vi "MCS.vi"(1 "MCS input":T1(array[cluster]) {"binning (s)" format="%.2f"; "binning (s)" format="%.2f"}, 2 "set":bool) -> (0 "MCS output":T1(array[cluster]) {"binning (s)" format="%.2f"; "binning (s)" format="%.2f"})   [LabVIEW 2009]
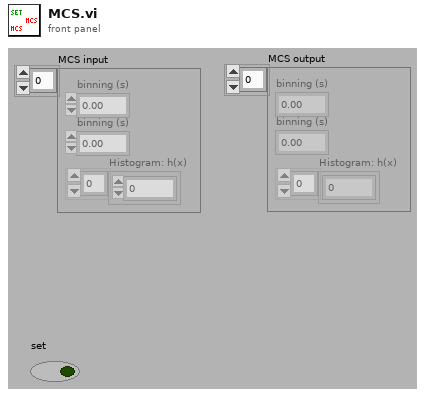
[diagram p1: front panel]
types:
  T1 = cluster{"binning (s)":dbl, "binning (s)":dbl, "Histogram: h(x)":u32[]}[]
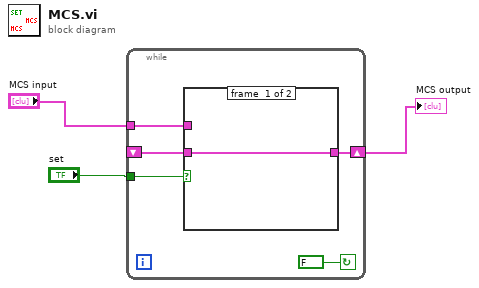
[diagram p0: block diagram]
diagram:
  n1 = while {
    shift-right: [w6] -> w1
    shift-left: _ -> [w4]
    tunnel: "set" -> [w7]
    tunnel: "MCS input" -> [w5]
    stop <- FALSE continue-if-true
    n2 = case shown="True" w7 {
      tunnel: [w9 w10] -> w6
      tunnel: w5 -> [_ w10]
      tunnel: w4 -> [w9 _]
      frame #0 {
      }
      frame #1 {
      }
    }
  }
  "MCS output" <- w1
